vi "FTW-Ether-Address-RandomEphemeral.vi"(5 "Endpoint":string, 11 "error in":errorcluster) -> (6 "Endpoint with Replacements":string, 15 "error out":errorcluster)   [LabVIEW 2013, in "FTW-Ether.lvclass"]
uses:
  FTW-Ether.lvclass
panel:
  # "Inputs"
  # "Outputs"
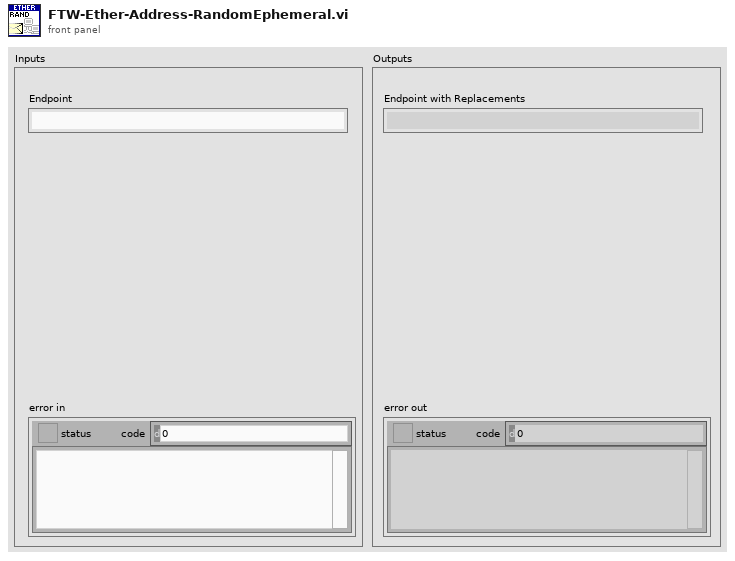
[diagram p1: front panel]
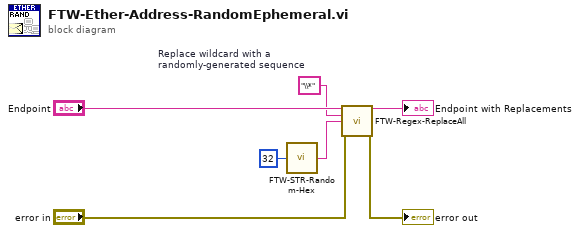
[diagram p0: block diagram]
diagram:
  w3 = "\\*"  # Replace wildcard with a randomly-generated sequence
  n1 = call "FTW-STR-Random-Hex.vi"("String Length"=32) -> ("Random Hex String"=w1:string)  [unwired: 3 in]
  n2 = call "FTW-Regex-ReplaceAll.vi"("String"="Endpoint", "Search for (Regular Expression)"=w3, "Replace with"=w1, "error in"="error in") -> ("String out"=→"Endpoint with Replacements":string, "error out"=→"error out":errorcluster)  [unwired: 9 in, 1 out]
